vi "Format Variant Into String Patched.vi"(0 "Input String":string, 2 "Format String":string, 7 "error in (no error)":errorcluster, 11 "Variant":variant) -> (4 "Output String":string, 8 "error out":errorcluster)   [LabVIEW 2015, in "LV String Utils v1.lvlib"]
doc: "Patched version of 'Format Variant Into String'. It supports %s and %d placeholders for enums giving access to names and values respectively."
uses:
  LV String Utils v1.lvlib
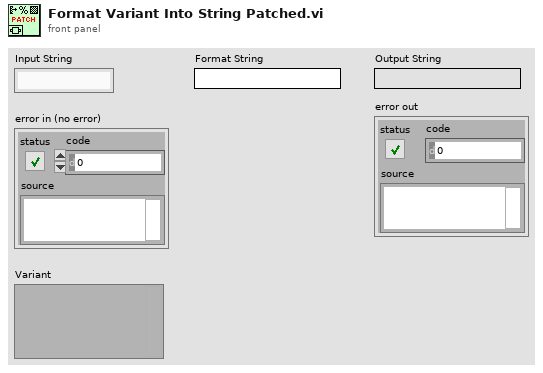
[diagram p1: front panel]
types:
  T1 = typedef "Type Descriptor Enumeration__ogtk.ctl" = enum8{"<Null>", "I8", "I16", "I32", "I64", "U8", "U16", "U32", "U64", "SGL", "DBL", "EXT", "CSG", "CDB", "CXT", "0x0F", "0x10", "0x11", "0x12", "0x13", "0x14", "Enum U8", "Enum U16", "Enum U32", "Enum U64", "SGL PQ", "DBL PQ", "EXT PQ", "CSG PQ", "CDB PQ", "CXT PQ", "0x1F", "0x20", "Boolean", "0x22", "0x23", "0x24", "0x25", "0x26", "0x27", "0x28", "0x29", "0x2A", "0x2B", "0x2C", "0x2D", "0x2E", "0x2F", "String", "0x31", "Path", "Pict", "0x34", "0x35", "0x36", "DAQ", "0x38", "0x39", "0x3A", "0x3B", "0x3C", "0x3D", "0x3E", "0x3F", "Array", "0x41", "0x42", "0x43", "0x44", "0x45", "0x46", "0x47", "0x48", "0x49", "0x4A", "0x4B", "0x4C", "0x4D", "0x4E", "0x4F", "Cluster", "0x51", "0x52", "Variant", "Waveform", "0x55", "0x56", "0x57", "0x58", "0x59", "0x5A", "0x5B", "0x5C", "0x5D", "0x5E", "0x5F", "0x60", "0x61", "0x62", "0x63", "0x64", "0x65", "0x66", "0x67", "0x68", "0x69", "0x6A", "0x6B", "0x6C", "0x6D", "0x6E", "0x6F", "Refnum"}
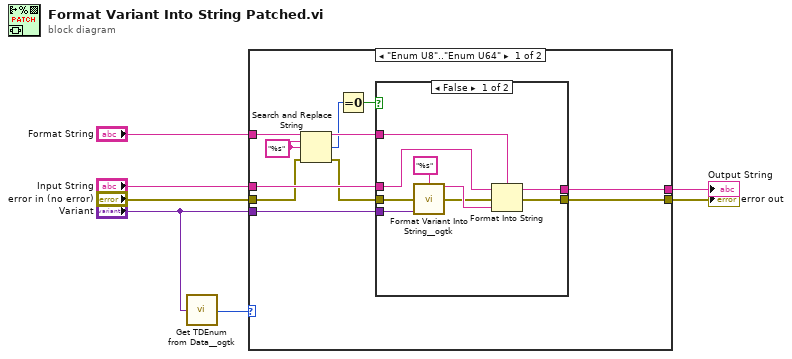
[diagram p0: block diagram]
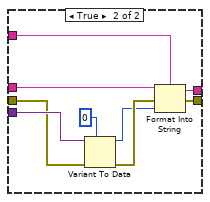
[diagram p2: hidden frame]
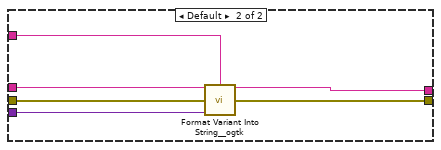
[diagram p3: hidden frame]
diagram:
  n1 = call <userlib>:"Get TDEnum from Data__ogtk.vi"("Data"="Variant") -> ("Type Descriptor Enumeration"=w2:T1)  [unwired: 4 in]
  n2 = case shown="\"Enum U8\"..\"Enum U64\"" w2 {
    tunnel: [w15 w42] -> w7
    tunnel: "error in (no error)" -> [w12 w41]
    tunnel: [w18 w40] -> w5
    tunnel: "Input String" -> [w17 w39]
    tunnel: "Variant" -> [w16 w38]
    tunnel: "Format String" -> [w14 w37]
    frame "Enum U8".."Enum U64" {
      w10 = "%s" ("search string")
      n3 = Search and Replace String(input string=w14, search string=w10, replace string=w10, error in=w12) -> (result string=w13:string, number of replacements=w9:i32, error out=w11:errorcluster)  [unwired: 4 in, 1 out]
      n4 = Equal To 0?(x=w9) -> (x = 0?=w8:bool)
      n5 = case shown="False" w8 {
        tunnel: [w19 w36] -> w18
        tunnel: w17 -> [w21 w35]
        tunnel: w16 -> [w25 w33]
        tunnel: w11 -> [w26 w32]
        tunnel: [w20 w29] -> w15
        tunnel: w13 -> [w24 w28]
        frame False {
          n6 = call <userlib>:"Format Variant Into String__ogtk.vi"("Format String"="%s", "error in (no error)"=w26, "Variant"=w25) -> ("Output String"=w23:string, "error out"=w22:errorcluster)  [unwired: 11 in]
          n7 = Format Into String(format string=w24, initial string=w21, error in=w22, w23) -> (resulting string=w20:string, error out=w19:errorcluster)
        }
        frame True {
          n8 = Variant To Data(error in=w32, type=u64 0, Variant=w33) -> (data=w30:u64, error out=w31:errorcluster)
          n9 = Format Into String(format string=w28, initial string=w35, error in=w31, w30) -> (resulting string=w29:string, error out=w36:errorcluster)
        }
      }
    }
    frame Default {
      n10 = call <userlib>:"Format Variant Into String__ogtk.vi"("Input String"=w39, "Format String"=w37, "error in (no error)"=w41, "Variant"=w38) -> ("Output String"=w42:string, "error out"=w40:errorcluster)  [unwired: 10 in]
    }
  }
  "Output String" <- w7
  "error out" <- w5
